vi "SubMatrixBias.vi"(0 "VgCluster":T1={"Target Bias, V"=1.0, "Sweep rate, V/min"=1.0, "Time btw \npoints, sec"=1.0, "points at each Vg"=1, "Set compliance limit, mkA"=0.05} {"Set compliance limit, mkA" min=0.0 max=1.0 step=0.01 format="%.3f"; "Time btw \npoints, sec" format="%.2f"; "Sweep rate, V/min" min=0.0 max=1.0 step=0.01 format="%.4f"; "Target Bias, V" min=-4.0 max=4.0 step=0.1 format="%.4f"}, 1 "Instruments":T3={"Oscillator"=TRUE, "Addr 1 lock-in"=TRUE, "Addr 1 lock-in oop"=TRUE, "Addr 2 lock-in"=FALSE, "Addr 2 lock-in oop"=FALSE, "Addr 3 lock-in"=FALSE, "Addr 3 lock-in oop"=FALSE, "Voltage (Vk1)"=FALSE, "Current (Ik1)"=TRUE, "Voltage (Vk2)"=FALSE, "Current (Ik2)"=FALSE, "Voltage (Vk3)"=FALSE, "Current (Ik3)"=FALSE, "Channel 1 (Vnano1)  "=FALSE, "Channel 2 (Vnano1b)"=FALSE, "Channel 1 (Vnano2)   "=FALSE, "Channel 2 (Vnano2b)"=FALSE, "Thermometer 1 (T1)"=TRUE, "Magnetic Field (B)"=TRUE, "Capacitance (C) and Loss (L)"=FALSE}, 2 "Settings":T2={"Ring 3"=1, "Ring 2"=4, "Fixed Current mkA"=0.5, "If yes, the current is:"=enum."Radio Selection 1", "Ressitance measurements?"=TRUE, "Commute DC current?"=FALSE} {"Ring 3" items=["1 kOhm", "10 kOhm", "100 kOhm", "1 Mohm", "10 mOhm"]; "Ring 2" items=["1 kOhm", "10 kOhm", "100 kOhm", "1 Mohm", "10 MOhm"]}, 3 "Custom Folder":string, 4 "Time Stamp":timestamp) -> ()   [LabVIEW 2015]
uses:
  <vilib>/Utility/file.llb/Write To Spreadsheet File (DBL).vi
panel:
  out "Current":dbl
  out "Comments":string[](array[string])
  out "ArrayBoolian":bool[][](array[boolean])
  out "Delib Time delay":i32
  out "XY Graph":cluster{dbl[], dbl[]}(graph)={[1.0, 0.8, 0.6000000000000001, 0.4000000000000001, 0.20000000000000007, 5.551115123125783e-17, -0.19999999999999996, -0.39999999999999997, -0.6, -0.8, -1.0], [0.03352775, 0.056811, 0.03911575, 0.04330675, -0.02468015, 0.011641600000000002, 0.10151450000000001, 0.12386675000000001, 0.08288825000000001, -0.00186266, -0.038650000000000004]}
  out "array for data":dbl[](array[numeric])
  in  "Ring":u16(ring) caption="Y-axis:" items=["Vg", "I", "R1", "R1oop", "Ik1", "T1", "B"]
  out "Data file:":path
  in  "error in (no error)":errorcluster
  # "Lock-in Amplifiers"
  # "Temperature"
  # "SourceMeters"
  # "Nanovoltmeters"
  # "Main"
  # "(not recommended, too slow)"
  # "Magnetic Field"
  # "Capacitance & Loss"
  # "(not recommended, too slow)"
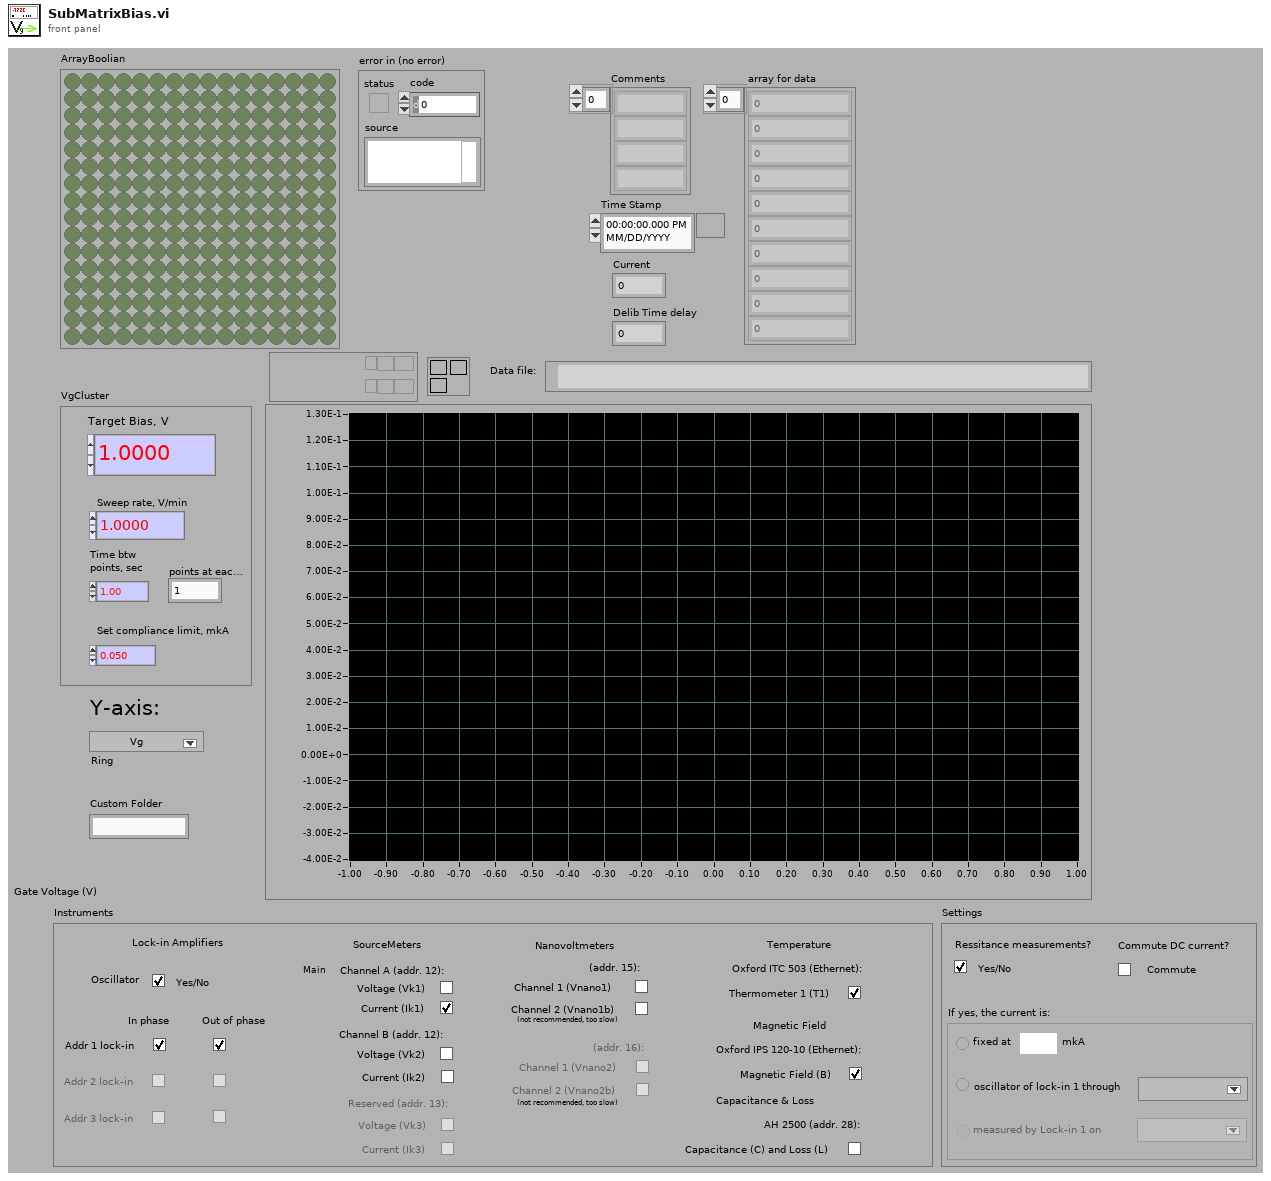
[diagram p1: front panel]
types:
  T1 = cluster{"Target Bias, V":dbl, "Sweep rate, V/min":dbl, "Time btw \npoints, sec":dbl, "points at each Vg":i32, "Set compliance limit, mkA":dbl}
  T2 = cluster{"Ring 3":u16, "Ring 2":u16, "Fixed Current mkA":dbl, "If yes, the current is:":enum32{"Radio Selection 1", "Radio Selection 2", "Radio Selection 3"}, "Ressitance measurements?":bool, "Commute DC current?":bool}
  T3 = cluster{"Oscillator":bool, "Addr 1 lock-in":bool, "Addr 1 lock-in oop":bool, "Addr 2 lock-in":bool, "Addr 2 lock-in oop":bool, "Addr 3 lock-in":bool, "Addr 3 lock-in oop":bool, "Voltage (Vk1)":bool, "Current (Ik1)":bool, "Voltage (Vk2)":bool, "Current (Ik2)":bool, "Voltage (Vk3)":bool, "Current (Ik3)":bool, "Channel 1 (Vnano1)  ":bool, "Channel 2 (Vnano1b)":bool, "Channel 1 (Vnano2)   ":bool, "Channel 2 (Vnano2b)":bool, "Thermometer 1 (T1)":bool, "Magnetic Field (B)":bool, "Capacitance (C) and Loss (L)":bool}
  T4 = enum32{"Radio Selection 1", "Radio Selection 2", "Radio Selection 3"}
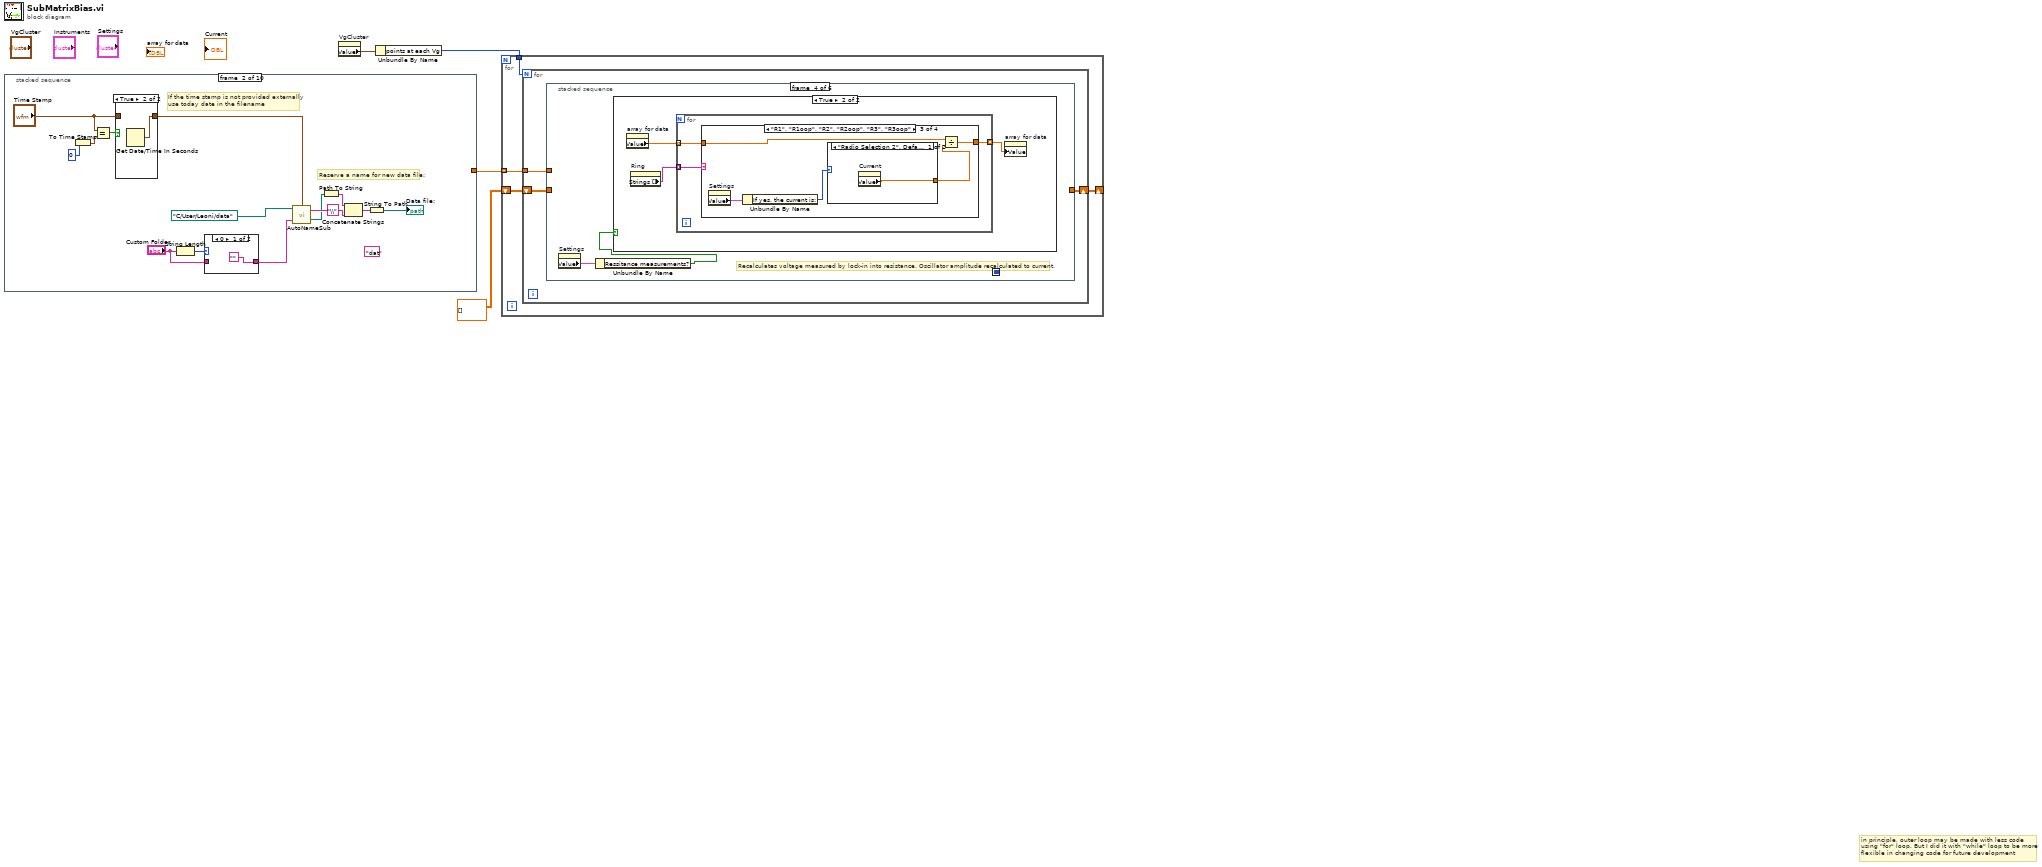
[diagram p0: block diagram]
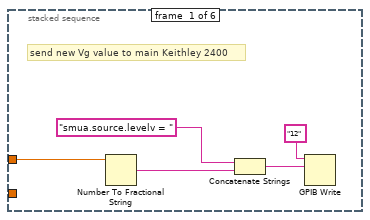
[diagram p2: hidden frame]
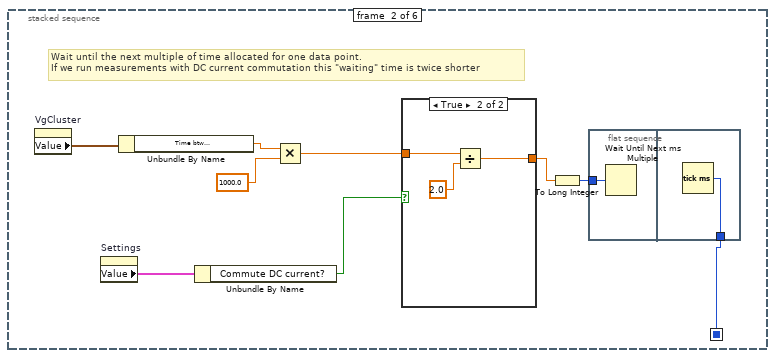
[diagram p3: hidden frame]
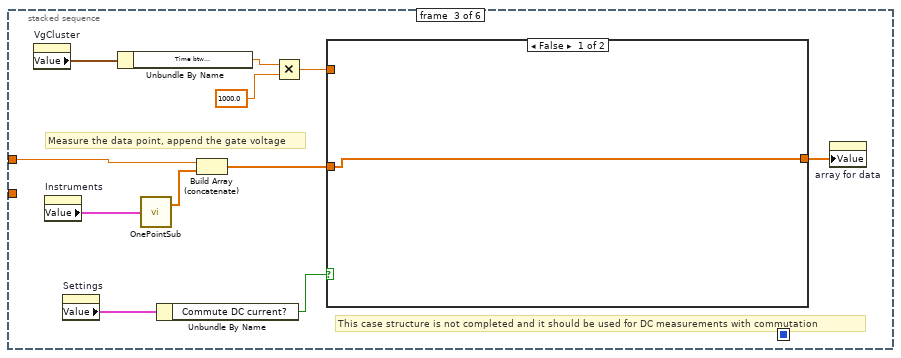
[diagram p5: hidden frame]
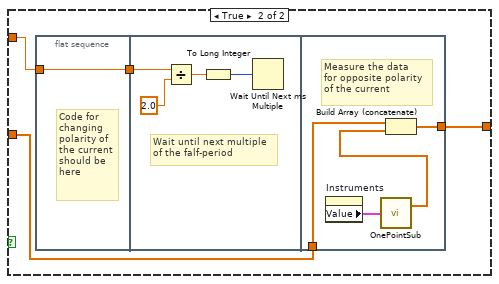
[diagram p6: hidden frame]
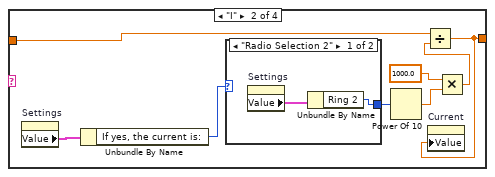
[diagram p9: hidden frame]
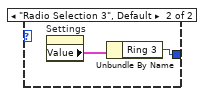
[diagram p10: hidden frame]
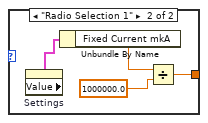
[diagram p11: hidden frame]
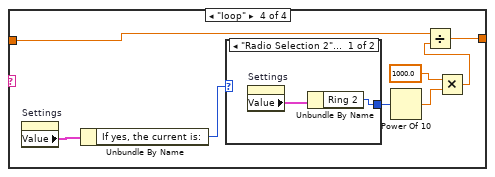
[diagram p12: hidden frame]
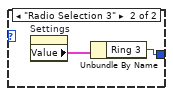
[diagram p13: hidden frame]
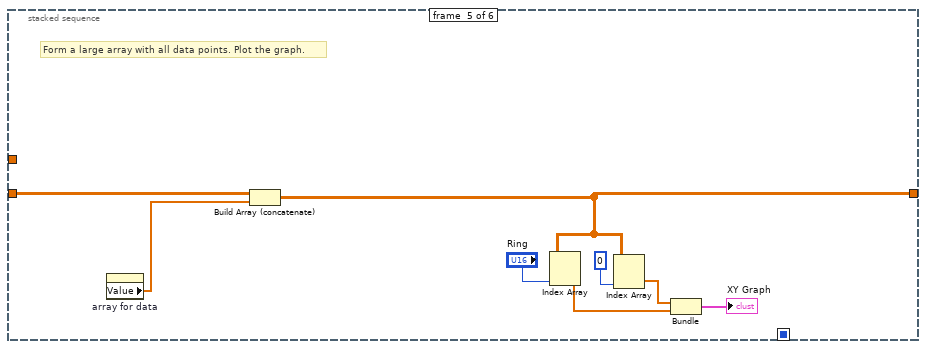
[diagram p14: hidden frame]
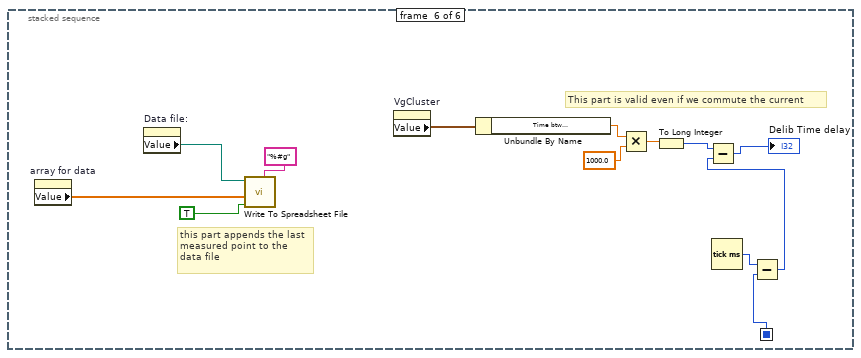
[diagram p15: hidden frame]
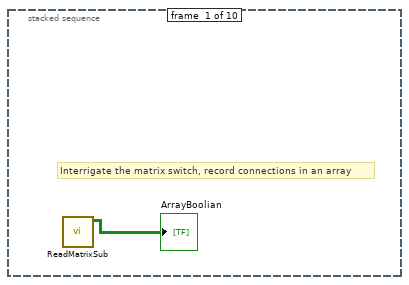
[diagram p16: hidden frame]
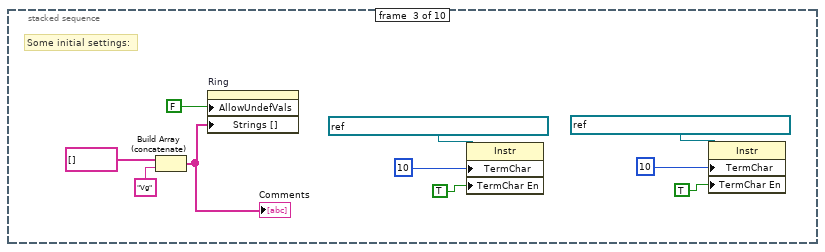
[diagram p19: hidden frame]
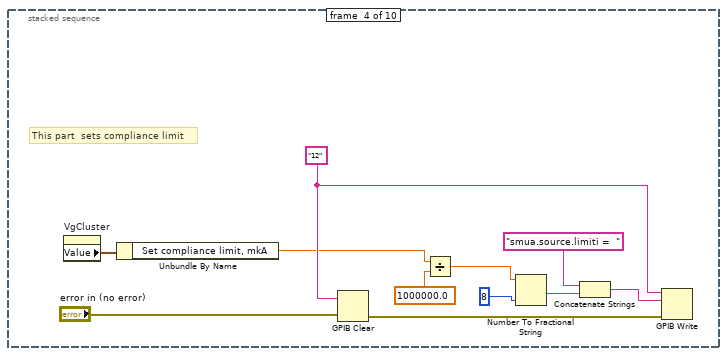
[diagram p20: hidden frame]
diagram:
  # "in principle, outer loop may be made with less code\nusing \"for\" loop. But I did it with \"while\" loop to be more \nflexible in changing code for future development"
  n1 = stacked-sequence {
    tunnel: [_ _ _ _ _ _ _ _ _ w125] -> w4
    frame #0 {
      # "Interrigate the matrix switch, record connections in an array"
      n2 = call "ReadMatrixSub.vi"() -> ("Array"=→"ArrayBoolian":bool[][])  [unwired: 9 in, 2 out]
    }
    frame #1 {
      (unwired) "dat"
      # "If the time stamp is not provided externally\nuse today date in the filename"
      # "Reserve a name for new data file:"
      n3 = To Time Stamp(1:0) -> (0:w9:timestamp)
      n4 = Equal?(x="Time Stamp", y=w9) -> (x = y?=w8:bool)
      n5 = case shown="True" w8 {
        tunnel: "Time Stamp" -> [w21 _]
        tunnel: [w21 w22] -> w6
        frame False {
        }
        frame True {
          n6 = Get Date/Time In Seconds() -> (seconds since 1Jan1904=w22:timestamp)
        }
      }
      n7 = String Length(string="Custom Folder") -> (length=w13:i32)
      n8 = case shown="0" w13 {
        tunnel: "Custom Folder" -> [_ w24]
        tunnel: ["" w24] -> w11
        frame 0 {
        }
        frame 1, Default {
        }
      }
      n9 = call "AutoNameSub.vi"("Time Stamp"=w6, "Custom Folder"=w11, "User Data Folder"=path "C:/User/Leoni/data") -> ("created path"=w19:path, "String"=w20:string)  [unwired: 1 in]
      n10 = Path To String(path=w19) -> (string=w14:string)
      n11 = Concatenate Strings(w14, "\\", w20) -> (w16:string)
      n12 = String To Path(string=w16) -> (path=→"Data file:":path)
    }
    frame #2 {
      # "Some initial settings:"
      n13 = Build Array (concatenate)(string[] [], "Vg") -> (w25:string[])
      "Comments" <- w25
      n14 = property on="Ring" class="Ring (strict)"("AllowUndefVals"=FALSE, "Strings []"=w25) -> ()  [unwired: 2 in, 2 out]
      n15 = property class="Instr"(reference=refnum<visa-resource-name> "TCPIP0::192.168.128.3::7020::SOCKET" ("VISA resource name"), "TermChar"=10, "TermChar En"=TRUE) -> ()  [unwired: 1 in, 2 out]
      n16 = property class="Instr"(reference=refnum<visa-resource-name> "TCPIP0::192.168.128.2::7020::SOCKET" ("VISA resource name"), "TermChar"=10, "TermChar En"=TRUE) -> ()  [unwired: 1 in, 2 out]
    }
    frame #3 {
      w38 = "12"
      # "This part  sets compliance limit"
      n17 = property on="VgCluster" class="Clust (strict)"() -> ("Value"=w36:T1)  [unwired: 2 in, 2 out]
      n18 = Unbundle By Name(w36) -> ("Set compliance limit, mkA"=w35:dbl)
      n19 = GPIB Clear(2:"error in (no error)", 3:w38) -> (0:w39:errorcluster)  [unwired: 1 out]
      n20 = Divide(x=w35, y=1000000.0) -> (x/y=w44:dbl)
      n21 = Number To Fractional String(number=w44, precision (6)=i16 8) -> (F-format string=w41:string)  [unwired: 2 in]
      n22 = Concatenate Strings("smua.source.limiti =  " ("data"), w41) -> (w40:string)
      n23 = GPIB Write(0:w38, 1:w40, 3:w39) -> ()  [unwired: 2 in, 2 out]
    }
    frame #4 {
      # "List of measured parameters obtained as \na text array and \"fed\" to a ring selector"
      # "When current is commutated every data point is measured twice (for both polarities of DC current). Names \nof parameters measured for negative polarity will start with lower case \"c\" (for \"commutated\")"
      # "Measurement of one data point (only to get the names of the parameters to be recorded)"
      n24 = property on="Settings" class="Clust (strict)"() -> ("Value"=w51:T2)  [unwired: 2 in, 2 out]
      n25 = property on="Instruments" class="Clust (strict)"() -> ("Value"=w49:T3)  [unwired: 2 in, 2 out]
      n26 = Unbundle By Name(w51) -> ("Commute DC current?"=w52:bool)
      n27 = call "OnePointSub.vi"("cluster"=w49) -> ("TextArray"=w50:string[])  [unwired: 2 in, 1 out]
      n28 = case shown="False" w52 {
        tunnel: w50 -> [w54 w61]
        tunnel: [w53 w61] -> w48
        frame True {
          n29 = for {
            tunnel: [w60] -> w57 mode=indexing
            tunnel: w54 -> [w58] mode=indexing
            n30 = Concatenate Strings("c", w58) -> (w60:string)
          }
          n31 = Array Subset(array=w57, index=1) -> (w55:string[])  [unwired: 1 in]
          n32 = Build Array (concatenate)(w54, w55) -> (w53:string[])
        }
        frame False {
        }
      }
      n33 = Build Array (concatenate)("Vg", w48) -> (w46:string[])
      n34 = property on="Ring" class="Ring (strict)"("Strings []"=w46) -> ()  [unwired: 2 in, 2 out]
    }
    frame #5 {
      # "If resistance is not something that we are interested in, then replace \"R\" with \"V\" in all strings"
      n35 = property on="Settings" class="Clust (strict)"() -> ("Value"=w62:T2)  [unwired: 2 in, 2 out]
      n36 = Unbundle By Name(w62) -> ("Ressitance measurements?"=w63:bool)
      n37 = case shown="False" w63 {
        frame True {
        }
        frame False {
          n38 = property on="Ring" class="Ring (strict)"() -> ("Strings []"=w65:string[])  [unwired: 2 in, 2 out]
          n39 = for {
            tunnel: w65 -> [w68] mode=indexing
            tunnel: [w66] -> w64 mode=indexing
            n40 = String Subset(string=w68, length (rest)=1) -> (substring=w70:string)  [unwired: 1 in]
            n41 = Equal?(x=w70, y="R") -> (x = y?=w69:bool)
            n42 = case shown="True" w69 {
              tunnel: w68 -> [w72 w76]
              tunnel: [w72 w73] -> w66
              frame False {
              }
              frame True {
                n43 = Replace Substring(2:1, 4:"V", 5:w76) -> (1:w73:string)  [unwired: 1 in, 1 out]
              }
            }
          }
          n44 = property on="Ring" class="Ring (strict)"("Strings []"=w64) -> ()  [unwired: 2 in, 2 out]
        }
      }
    }
    frame #6 {
      # "This part makes comment line for the \ndata file. Comments are very useful for\ndouble checking that connections are \ncorrect when the data file is opened\nin Origin."
      # "Check how the oscillator is wired to the matrix switch and record connection as a comment"
      n45 = property on="Instruments" class="Clust (strict)"() -> ("Value"=w79:T3)  [unwired: 2 in, 2 out]
      n46 = property on="Comments" class="Arr (strict)"() -> ("Value"=w78:string[])  [unwired: 2 in, 2 out]
      n47 = Unbundle By Name(w79) -> ("Oscillator"=w80:bool)
      n48 = case shown="True" w80 {
        tunnel: [w81 w84] -> w77
        tunnel: w78 -> [w81 w83]
        frame False {
          # "we are not measuring oscillator from\nlock-in (address 1)"
        }
        frame True {
          (unwired) "I"
          # "This subVI takes the matrix column # (instrument\nconnection point) as an argument and finds the raw\n# (contact) to which the instrument is connected"
          # "we are  measuring oscillator"
          n49 = property on="ArrayBoolian" class="Arr (strict)"() -> ("Value"=w87:bool[][])  [unwired: 2 in, 2 out]
          n50 = GPIB Clear(3:"1") -> ()  [unwired: 1 in, 2 out]
          n51 = call "FindInstrConnect.vi"("Column #"=1, "ArrayBoolian"=w87) -> ("String"=w88:string)  [unwired: 1 in, 2 out]
          n52 = call "FindInstrConnect.vi"("Column #"=0, "ArrayBoolian"=w87) -> ("String"=w85:string)  [unwired: 1 in, 2 out]
          n53 = Concatenate Strings(w85, "-", w88) -> (w82:string)
          n54 = Build Array (concatenate)(w83, w82) -> (w84:string[])
        }
      }
      n55 = property on="Comments" class="Arr (strict)"("Value"=w77) -> ()  [unwired: 2 in, 2 out]
    }
    frame #7 {
      # "Check how the input of Lock-in 1 is wired the the matrix switch and record connection as a comment"
      n56 = property on="Instruments" class="Clust (strict)"() -> ("Value"=w94:T3)  [unwired: 2 in, 2 out]
      n57 = property on="Comments" class="Arr (strict)"() -> ("Value"=w93:string[])  [unwired: 2 in, 2 out]
      n58 = Unbundle By Name(w94) -> ("Addr 1 lock-in"=w95:bool)
      n59 = case shown="True" w95 {
        tunnel: [w96 w99] -> w92
        tunnel: w93 -> [w96 w98]
        frame False {
          # "we are not measuring oscillator from\nlock-in (address 1)"
        }
        frame True {
          (unwired) "I"
          # "This subVI takes the matrix column # (instrument\nconnection point) as an argument and finds the raw\n# (contact) to which the instrument is connected"
          # "we are  measuring Lock-In 1"
          n60 = property on="ArrayBoolian" class="Arr (strict)"() -> ("Value"=w102:bool[][])  [unwired: 2 in, 2 out]
          n61 = GPIB Clear(3:"1") -> ()  [unwired: 1 in, 2 out]
          n62 = call "FindInstrConnect.vi"("Column #"=3, "ArrayBoolian"=w102) -> ("String"=w103:string)  [unwired: 1 in, 2 out]
          n63 = call "FindInstrConnect.vi"("Column #"=2, "ArrayBoolian"=w102) -> ("String"=w100:string)  [unwired: 1 in, 2 out]
          n64 = Concatenate Strings(w100, "-", w103) -> (w97:string)
          n65 = Build Array (concatenate)(w98, w97) -> (w99:string[])
        }
      }
      n66 = property on="Comments" class="Arr (strict)"("Value"=w92) -> ()  [unwired: 2 in, 2 out]
    }
    frame #8 {
      w115 = "\r"
      w114 = "\n"
      # "Both lines are recorded into\nthe data file."
      # "This part converts string array with the names of measured parameters into the line of text separated by TABs. The resulting string is\nrecorded as the first line of the data file. The second line is comments with information about conections of the instruments to particular contacts."
      n67 = property on="Ring" class="Ring (strict)"() -> ("Strings []"=w108:string[])  [unwired: 2 in, 2 out]
      n68 = property on="Comments" class="Arr (strict)"() -> ("Value"=w113:string[])  [unwired: 2 in, 2 out]
      n69 = for {
        tunnel: w108 -> [w123] mode=indexing
        shift-right: [w121] -> w111
        shift-left: "" -> [w122]
        n70 = Concatenate Strings(w122, w123, "\t") -> (w121:string)
      }
      n71 = for {
        tunnel: w113 -> [w119] mode=indexing
        shift-right: [w117] -> w116
        shift-left: "" -> [w118]
        n72 = Concatenate Strings(w118, w119, "\t") -> (w117:string)
      }
      n73 = Concatenate Strings(w111, w115, w114, w115, w114, w116, w115, w114) -> (w109:string)
      n74 = property on="Data file:" class="Path"() -> ("Value"=w107:path)  [unwired: 2 in, 2 out]
      n75 = Write to Text File(file (use dialog)=w107, text=w109) -> ()  [unwired: 2 in, 3 out]
    }
    frame #9 {
      w139 = "12"
      # "Then the table is made with all values\nof the gate voltage to be measured"
      # "rounding to 0.1 V"
      # "This part reads the output voltage on channel A of the main Keithly 2614B \n(address 12)"
      n76 = property on="VgCluster" class="Clust (strict)"() -> ("Value"=w133:T1)  [unwired: 2 in, 2 out]
      n77 = Unbundle By Name(w133) -> ("Target Bias, V"=w127:dbl, "Sweep rate, V/min"=w132:dbl, "Time btw \npoints, sec"=w131:dbl)
      n78 = GPIB Write(0:w139, 1:"print(smua.measure.v())" ("data")) -> (6:w142:errorcluster)  [unwired: 3 in, 1 out]
      n79 = GPIB Read(0:w139, 1:200 ("byte count"), 3:w142) -> (5:w134:string)  [unwired: 2 in, 2 out]
      n80 = Fract/Exp String To Number(string=w134) -> (number=w138:dbl)  [unwired: 3 in, 1 out]
      n81 = Multiply(x=w132, y=w131) -> (x*y=w130:dbl)
      n82 = Divide(x=w130, y=60.0) -> (x/y=w126:dbl)
      n83 = Number To Fractional String(number=w138, width (-)=5, precision (6)=1) -> (F-format string=w135:string)  [unwired: 1 in]
      n84 = Fract/Exp String To Number(string=w135) -> (number=w128:dbl)  [unwired: 3 in, 1 out]
      n85 = call "LinTableSubVI.vi"("Step"=w126, "Final"=w127, "Initial"=w128) -> ("Array"=w125:dbl[])  [unwired: 1 in]
    }
  }
  n86 = property on="VgCluster" class="Clust (strict)"() -> ("Value"=w3:T1)  [unwired: 2 in, 2 out]
  n87 = Unbundle By Name(w3) -> ("points at each Vg"=w2:i32)
  n88 = for {
    tunnel: w4 -> [w146] mode=indexing
    tunnel: w2 -> [w145]
    shift-right: [w143] -> _
    shift-left: dbl[][] [] -> [w144]
    n89 = for {
      N: w145 -> [_]
      tunnel: w146 -> [w149]
      shift-right: [w147] -> w143
      shift-left: w144 -> [w148]
      n90 = stacked-sequence {
        seq-local: [_ w155 _ _ _ _] -> [_ _ _ _ _ w253]
        tunnel: w149 -> [w151 _ w172 _ _ _]
        tunnel: w148 -> [_ _ _ _ w240 _]
        tunnel: [_ _ _ _ w238 _] -> w147
        frame #0 {
          # "send new Vg value to main Keithley 2400"
          n91 = Number To Fractional String(number=w151) -> (F-format string=w153:string)  [unwired: 3 in]
          n92 = Concatenate Strings("smua.source.levelv = " ("data"), w153) -> (w152:string)
          n93 = GPIB Write(0:"12", 1:w152) -> ()  [unwired: 3 in, 2 out]
        }
        frame #1 {
          # "Wait until the next multiple of time allocated for one data point.\nIf we run measurements with DC current commutation this \"waiting\" time is twice shorter"
          n94 = property on="VgCluster" class="Clust (strict)"() -> ("Value"=w163:T1)  [unwired: 2 in, 2 out]
          n95 = property on="Settings" class="Clust (strict)"() -> ("Value"=w160:T2)  [unwired: 2 in, 2 out]
          n96 = Unbundle By Name(w163) -> ("Time btw \npoints, sec"=w162:dbl)
          n97 = Unbundle By Name(w160) -> ("Commute DC current?"=w159:bool)
          n98 = Multiply(x=w162, y=1000.0) -> (x*y=w158:dbl)
          n99 = case shown="True" w159 {
            tunnel: w158 -> [w166 w168]
            tunnel: [w166 w167] -> w157
            frame False {
            }
            frame True {
              n100 = Divide(x=w168, y=2.0) -> (x/y=w167:dbl)
            }
          }
          n101 = To Long Integer(number=w157) -> (32bit integer=w156:i32)
          n102 = flat-sequence {
            tunnel: w156 -> [w164]
            tunnel: [w165] -> w155
            frame #0 {
              n103 = Wait Until Next ms Multiple(millisecond multiple=w164) -> ()  [unwired: 1 out]
            }
            frame #1 {
              n104 = Tick Count (ms)() -> (millisecond timer value=w165:u32)
            }
          }
        }
        frame #2 {
          # "This case structure is not completed and it should be used for DC measurements with commutation"
          # "Measure the data point, append the gate voltage"
          n105 = property on="VgCluster" class="Clust (strict)"() -> ("Value"=w180:T1)  [unwired: 2 in, 2 out]
          n106 = property on="Instruments" class="Clust (strict)"() -> ("Value"=w174:T3)  [unwired: 2 in, 2 out]
          n107 = property on="Settings" class="Clust (strict)"() -> ("Value"=w177:T2)  [unwired: 2 in, 2 out]
          n108 = Unbundle By Name(w180) -> ("Time btw \npoints, sec"=w179:dbl)
          n109 = call "OnePointSub.vi"("cluster"=w174) -> ("Array"=w173:dbl[])  [unwired: 2 in, 1 out]
          n110 = Unbundle By Name(w177) -> ("Commute DC current?"=w176:bool)
          n111 = Build Array (concatenate)(w172, w173) -> (w171:dbl[])
          n112 = Multiply(x=w179, y=1000.0) -> (x*y=w175:dbl)
          n113 = case shown="False" w176 {
            tunnel: w175 -> [_ w185]
            tunnel: [w181 w182] -> w170
            tunnel: w171 -> [w181 w183]
            frame False {
            }
            frame True {
              n114 = flat-sequence {
                tunnel: w185 -> [w186]
                tunnel: [w186] -> w184
                tunnel: w184 -> [w189]
                tunnel: w183 -> [w192]
                tunnel: [w191] -> w182
                frame #0 {
                  # "Code for \nchanging \npolarity of \nthe current\nshould be \nhere"
                }
                frame #1 {
                  # "Wait until next multiple\nof the falf-period"
                  n115 = Divide(x=w189, y=2.0) -> (x/y=w187:dbl)
                  n116 = To Long Integer(number=w187) -> (32bit integer=w188:i32)
                  n117 = Wait Until Next ms Multiple(millisecond multiple=w188) -> ()  [unwired: 1 out]
                }
                frame #2 {
                  # "Measure the data\nfor opposite polarity\nof the current"
                  n118 = property on="Instruments" class="Clust (strict)"() -> ("Value"=w194:T3)  [unwired: 2 in, 2 out]
                  n119 = call "OnePointSub.vi"("cluster"=w194) -> ("Array"=w193:dbl[])  [unwired: 2 in, 1 out]
                  n120 = Build Array (concatenate)(w192, w193) -> (w191:dbl[])
                }
              }
            }
          }
          n121 = property on="array for data" class="Arr (strict)"("Value"=w170) -> ()  [unwired: 2 in, 2 out]
        }
        frame #3 {
          # "Recalculates voltage measured by lock-in into resistance. Oscillator amplitude recalculated to current."
          n122 = property on="Settings" class="Clust (strict)"() -> ("Value"=w196:T2)  [unwired: 2 in, 2 out]
          n123 = Unbundle By Name(w196) -> ("Ressitance measurements?"=w195:bool)
          n124 = case shown="True" w195 {
            frame False {
            }
            frame True {
              n125 = property on="array for data" class="Arr (strict)"() -> ("Value"=w198:dbl[])  [unwired: 2 in, 2 out]
              n126 = property on="Ring" class="Ring (strict)"() -> ("Strings []"=w199:string[])  [unwired: 2 in, 2 out]
              n127 = for {
                tunnel: w199 -> [w202] mode=indexing
                tunnel: w198 -> [w201] mode=indexing
                tunnel: [w200] -> w197 mode=indexing
                n128 = case shown="\"R1\", \"R1oop\", \"R2\", \"R2oop\", \"R3\", \"R3oop\"" w202 {
                  tunnel: w201 -> [w203 w206 w218 w228]
                  tunnel: [w203 w204 w217 w227] -> w200
                  frame "False", Default {
                  }
                  frame "I" {
                    n129 = property on="Settings" class="Clust (strict)"() -> ("Value"=w211:T2)  [unwired: 2 in, 2 out]
                    n130 = Unbundle By Name(w211) -> ("If yes, the current is:"=w210:T4)
                    n131 = case shown="\"Radio Selection 2\"" w210 {
                      tunnel: [w212 w214] -> w205
                      frame "Radio Selection 2" {
                        n132 = property on="Settings" class="Clust (strict)"() -> ("Value"=w213:T2)  [unwired: 2 in, 2 out]
                        n133 = Unbundle By Name(w213) -> ("Ring 2"=w212:u16)
                      }
                      frame "Radio Selection 3", Default {
                        n134 = property on="Settings" class="Clust (strict)"() -> ("Value"=w215:T2)  [unwired: 2 in, 2 out]
                        n135 = Unbundle By Name(w215) -> ("Ring 3"=w214:u16)
                      }
                    }
                    n136 = Power Of 10(x=w205) -> (10^x=w209:dbl)
                    n137 = Multiply(x=1000.0, y=w209) -> (x*y=w207:dbl)
                    n138 = Divide(x=w206, y=w207) -> (x/y=w204:dbl)
                    n139 = property on="Current" class="DigNum (strict)"("Value"=w204) -> ()  [unwired: 2 in, 2 out]
                  }
                  frame "R1", "R1oop", "R2", "R2oop", "R3", "R3oop" {
                    n140 = property on="Settings" class="Clust (strict)"() -> ("Value"=w220:T2)  [unwired: 2 in, 2 out]
                    n141 = Unbundle By Name(w220) -> ("If yes, the current is:"=w219:T4)
                    n142 = case shown="\"Radio Selection 2\", Default" w219 {
                      tunnel: [w221 w224] -> w216
                      frame "Radio Selection 2", Default {
                        n143 = property on="Current" class="DigNum (strict)"() -> ("Value"=w221:dbl)  [unwired: 2 in, 2 out]
                      }
                      frame "Radio Selection 1" {
                        n144 = property on="Settings" class="Clust (strict)"() -> ("Value"=w225:T2)  [unwired: 2 in, 2 out]
                        n145 = Unbundle By Name(w225) -> ("Fixed Current mkA"=w223:dbl)
                        n146 = Divide(x=w223, y=1000000.0) -> (x/y=w224:dbl)
                      }
                    }
                    n147 = Divide(x=w218, y=w216) -> (x/y=w217:dbl)
                  }
                  frame "Ioop" {
                    n148 = property on="Settings" class="Clust (strict)"() -> ("Value"=w233:T2)  [unwired: 2 in, 2 out]
                    n149 = Unbundle By Name(w233) -> ("If yes, the current is:"=w232:T4)
                    n150 = case shown="\"Radio Selection 2\", Default" w232 {
                      tunnel: [w234 w236] -> w226
                      frame "Radio Selection 2", Default {
                        n151 = property on="Settings" class="Clust (strict)"() -> ("Value"=w235:T2)  [unwired: 2 in, 2 out]
                        n152 = Unbundle By Name(w235) -> ("Ring 2"=w234:u16)
                      }
                      frame "Radio Selection 3" {
                        n153 = property on="Settings" class="Clust (strict)"() -> ("Value"=w237:T2)  [unwired: 2 in, 2 out]
                        n154 = Unbundle By Name(w237) -> ("Ring 3"=w236:u16)
                      }
                    }
                    n155 = Power Of 10(x=w226) -> (10^x=w231:dbl)
                    n156 = Multiply(x=1000.0, y=w231) -> (x*y=w229:dbl)
                    n157 = Divide(x=w228, y=w229) -> (x/y=w227:dbl)
                  }
                }
              }
              n158 = property on="array for data" class="Arr (strict)"("Value"=w197) -> ()  [unwired: 2 in, 2 out]
            }
          }
        }
        frame #4 {
          # "Form a large array with all data points. Plot the graph."
          n159 = property on="array for data" class="Arr (strict)"() -> ("Value"=w239:dbl[])  [unwired: 2 in, 2 out]
          n160 = Build Array (concatenate)(w240, w239) -> (w238:dbl[][])
          n161 = Index Array(array=w238, index (col)="Ring") -> (element=w245:dbl[])  [unwired: 1 in]
          n162 = Index Array(array=w238, index (col)=0) -> (element=w243:dbl[])  [unwired: 1 in]
          n163 = Bundle(w243, w245) -> (→"XY Graph":cluster{dbl[], dbl[]})  [unwired: 1 in]
        }
        frame #5 {
          # "This part is valid even if we commute the current"
          # "this part appends the last\nmeasured point to the \ndata file"
          n164 = property on="array for data" class="Arr (strict)"() -> ("Value"=w258:dbl[])  [unwired: 2 in, 2 out]
          n165 = property on="Data file:" class="Path"() -> ("Value"=w256:path)  [unwired: 2 in, 2 out]
          n166 = call-poly <vilib>:"Write To Spreadsheet File.vi"("format (%.3f)"="%#g", "append to file? (new file:F)"=TRUE, "1D data"=w258, "file path (dialog if empty)"=w256) -> ()  [unwired: 4 in, 1 out]
          n167 = property on="VgCluster" class="Clust (strict)"() -> ("Value"=w252:T1)  [unwired: 2 in, 2 out]
          n168 = Unbundle By Name(w252) -> ("Time btw \npoints, sec"=w251:dbl)
          n169 = Multiply(x=w251, y=1000.0) -> (x*y=w249:dbl)
          n170 = To Long Integer(number=w249) -> (32bit integer=w248:i32)
          n171 = Tick Count (ms)() -> (millisecond timer value=w254:u32)
          n172 = Subtract(x=w254, y=w253) -> (x-y=w246:u32)
          n173 = Subtract(x=w248, y=w246) -> (x-y=→"Delib Time delay":u32)
        }
      }
    }
  }
